vi "Set Control Values.vi"(8 "error in (no error)":errorcluster, 10 "Control References":T1, 11 "node in":refnum<class "RIO Target.lvclass">) -> (0 "error out":errorcluster, 3 "node out":refnum<class "RIO Target.lvclass">)   [LabVIEW 2014, in "RIO Target.lvclass"]
uses:
  RIO Target.lvclass
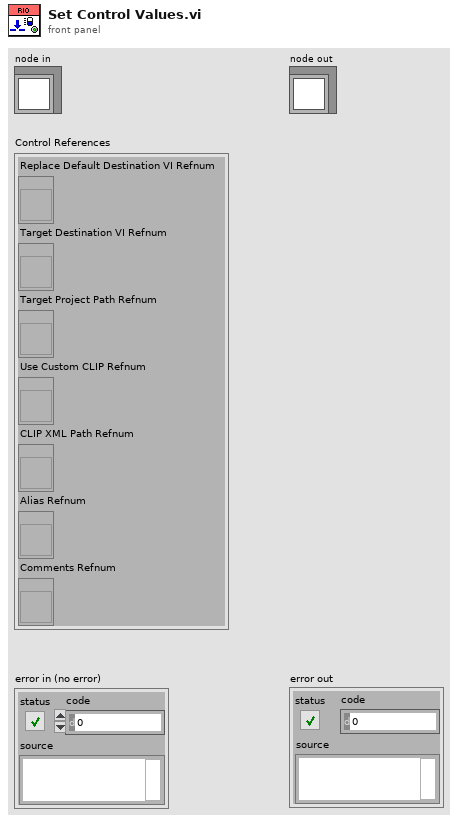
[diagram p1: front panel]
types:
  T1 = cluster{"Replace Default Destination VI Refnum":refnum<vi>, "Target Destination VI Refnum":refnum<vi>, "Target Project Path Refnum":refnum<vi>, "Use Custom CLIP Refnum":refnum<vi>, "CLIP XML Path Refnum":refnum<vi>, "Alias Refnum":refnum<vi>, "Comments Refnum":refnum<vi>}
  T2 = typedef "RIO Target.lvclass/UI Configuration.ctl" = cluster{"Destination VI":path, "Target Project Path":path, "CLIP XML Path":path, "Alias":string, "Comments":string, "Replace Default VI?":bool, "Use Custom CLIP?":bool}
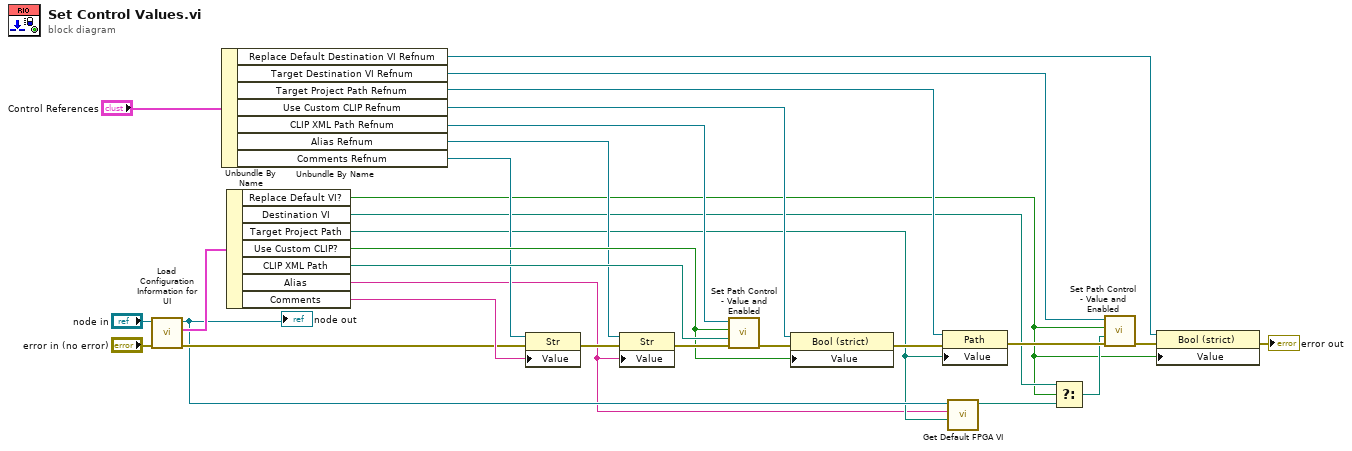
[diagram p0: block diagram]
diagram:
  n1 = call "Load Configuration Information for UI.vi"("error in (no error)"="error in (no error)", "node in"="node in") -> ("error out"=w11:errorcluster, "UI Configuration"=w29:T2, "node out"=w7:refnum<class "RIO Target.lvclass">)  [unwired: 7 in]
  "node out" <- w7
  n2 = Unbundle By Name("Control References") -> ("Replace Default Destination VI Refnum"=w18:refnum<vi>, "Target Destination VI Refnum"=w17:refnum<vi>, "Target Project Path Refnum"=w16:refnum<vi>, "Use Custom CLIP Refnum"=w15:refnum<vi>, "CLIP XML Path Refnum"=w14:refnum<vi>, "Alias Refnum"=w13:refnum<vi>, "Comments Refnum"=w12:refnum<vi>)
  n3 = Unbundle By Name(w29) -> ("Replace Default VI?"=w1:bool, "Destination VI"=w3:path, "Target Project Path"=w6:path, "Use Custom CLIP?"=w21:bool, "CLIP XML Path"=w25:path, "Alias"=w5:string, "Comments"=w27:string)
  n4 = property class="Str"(reference=w12, error in=w11, "Value"=w27) -> (error out=w28:errorcluster)  [unwired: 1 out]
  n5 = property class="Str"(reference=w13, error in=w28, "Value"=w5) -> (error out=w26:errorcluster)  [unwired: 1 out]
  n6 = call "Set Path Control - Value and Enabled.vi"("error in (no error)"=w26, "Value"=w25, "Enabled?"=w21, "Path in"=w14) -> ("error out"=w23:errorcluster)  [unwired: 7 in]
  n7 = property class="Bool (strict)"(reference=w15, error in=w23, "Value"=w21) -> (error out=w20:errorcluster)  [unwired: 1 out]
  n8 = property class="Path"(reference=w16, error in=w20, "Value"=w6) -> (error out=w24:errorcluster)  [unwired: 1 out]
  n9 = call "Get Default FPGA VI.vi"("Target Project Path"=w6, "Alias"=w5, "LabVIEW Object in"=w7) -> ("appended path"=w4:path)  [unwired: 8 in]
  n10 = Select(t=w3, s=w1, f=w4) -> (s? t:f=w2:path)
  n11 = call "Set Path Control - Value and Enabled.vi"("error in (no error)"=w24, "Value"=w2, "Enabled?"=w1, "Path in"=w17) -> ("error out"=w22:errorcluster)  [unwired: 7 in]
  n12 = property class="Bool (strict)"(reference=w18, error in=w22, "Value"=w1) -> (error out=→"error out":errorcluster)  [unwired: 1 out]
